vi "Volt_to_Temp.vi"(1 "Voltage":dbl) -> (0 "Temperature":dbl)   [LabVIEW 2010]
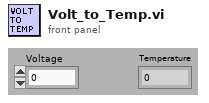
[diagram p1: front panel]
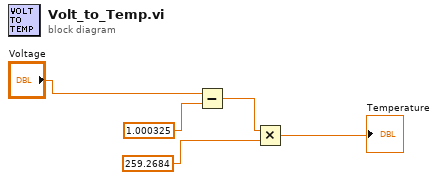
[diagram p0: block diagram]
diagram:
  n1 = Subtract(x="Voltage", y=1.000325) -> (x-y=w3:dbl)
  n2 = Multiply(x=w3, y=259.2684) -> (x*y=→"Temperature":dbl)
